vi "Auto_Routine_DepositConeBalance.vi"(8 "error in (no error)":errorcluster, 11 "IsBlue?":bool) -> (0 "error out":errorcluster)   [LabVIEW 2023]
doc: "deposits cone, drives backwards, balances. Starts from 3rd node from non pickup edge. Determines is it is blue or red (by IsBlue?) then changes actions accordingly.\n\ninputs: \n--IsBlue?--Boolean--\n--ErrorIn--\noutputs:\n--ErrorOut--"
uses:
  Arm/ArmGamePiecePreset.ctl
  Arm/ArmPositionPreset.ctl
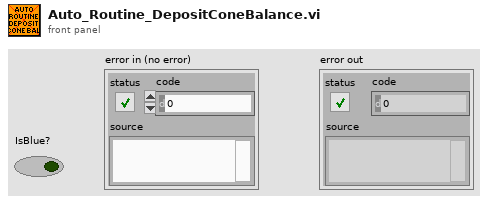
[diagram p1: front panel]
types:
  T1 = typedef "ArmGamePiecePreset.ctl" = enum16{"Cube", "Cone"}
  T2 = typedef "ArmPositionPreset.ctl" = enum16{"Upper", "Lower", "Middle", "Home", "Shelf", "Floor", "HalfFloor", "HalfHome"}
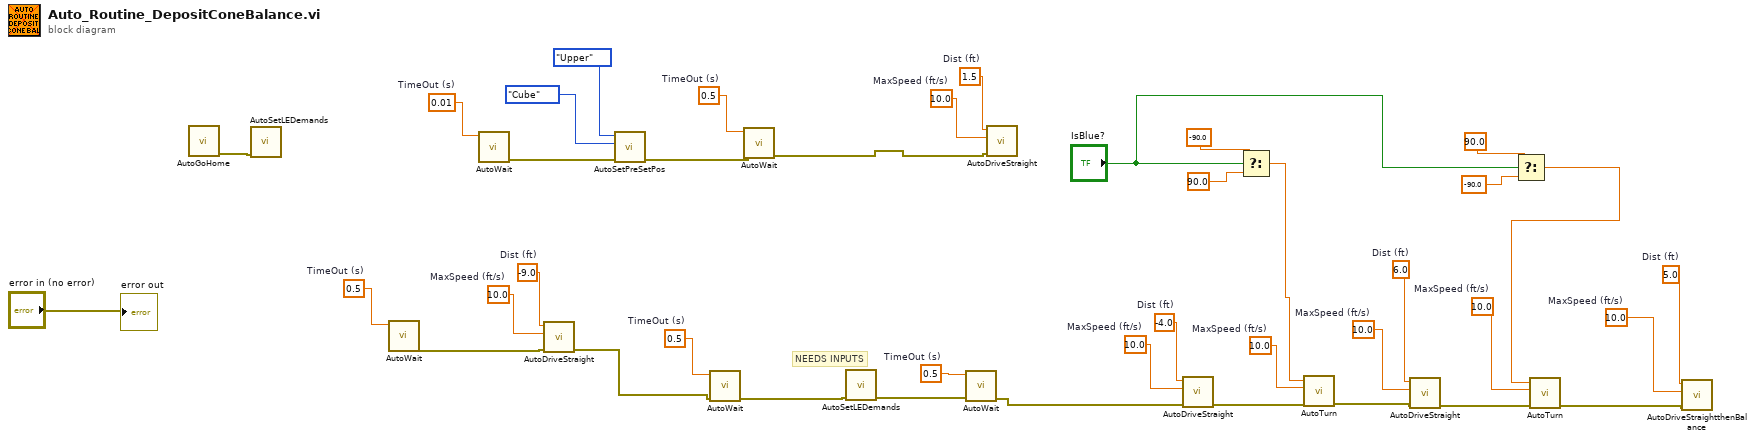
[diagram p0: block diagram]
diagram:
  w14 = 10.0  # MaxSpeed (ft/s)
  w15 = 5.0  # Dist (ft)
  w18 = 10.0  # MaxSpeed (ft/s)
  w19 = 10.0  # MaxSpeed (ft/s)
  w20 = 6.0  # Dist (ft)
  w22 = 10.0  # MaxSpeed (ft/s)
  w24 = -4.0  # Dist (ft)
  w25 = 10.0  # MaxSpeed (ft/s)
  w27 = 0.5  # TimeOut (s)
  w29 = 0.5  # TimeOut (s)
  w31 = -9.0  # Dist (ft)
  w32 = 10.0  # MaxSpeed (ft/s)
  w33 = 0.5  # TimeOut (s)
  w34 = 1.5  # Dist (ft)
  w35 = 10.0  # MaxSpeed (ft/s)
  w37 = 0.5  # TimeOut (s)
  w39 = 0.01  # TimeOut (s)
  # "NEEDS INPUTS"
  n1 = call "AutoGoHome.vi"() -> ("error out"=w1:errorcluster)  [unwired: 11 in]
  n2 = call "AutoSetLEDemands.vi"("error in (no error)"=w1) -> ()  [unwired: 10 in, 1 out]
  n3 = call "AutoWait.vi"("TimeOut (s)"=w33) -> ("error out"=w30:errorcluster)  [unwired: 10 in]
  n4 = call "AutoWait.vi"("TimeOut (s)"=w39) -> ("error out"=w38:errorcluster)  [unwired: 10 in]
  n5 = call "AutoDriveStraight.vi"("error in (no error)"=w30, "MaxSpeed (ft/s)"=w32, "Dist (ft)"=w31) -> ("error out"=w11:errorcluster)  [unwired: 8 in]
  n6 = call "AutoSetPreSetPos.vi"("error in (no error)"=w38, "Game Piece"=ArmGamePiecePreset."Cube", "Position"=ArmPositionPreset."Upper") -> ("error out"=w36:errorcluster)  [unwired: 8 in]
  n7 = call "AutoWait.vi"("error in (no error)"=w11, "TimeOut (s)"=w29) -> ("error out"=w28:errorcluster)  [unwired: 9 in]
  n8 = call "AutoWait.vi"("error in (no error)"=w36, "TimeOut (s)"=w37) -> ("error out"=w10:errorcluster)  [unwired: 9 in]
  n9 = call "AutoSetLEDemands.vi"("error in (no error)"=w28) -> ("error out"=w26:errorcluster)  [unwired: 10 in]
  n10 = call "AutoWait.vi"("error in (no error)"=w26, "TimeOut (s)"=w27) -> ("error out"=w9:errorcluster)  [unwired: 9 in]
  n11 = call "AutoDriveStraight.vi"("error in (no error)"=w10, "MaxSpeed (ft/s)"=w35, "Dist (ft)"=w34) -> ()  [unwired: 8 in, 1 out]
  n12 = call "AutoDriveStraight.vi"("error in (no error)"=w9, "MaxSpeed (ft/s)"=w25, "Dist (ft)"=w24) -> ("error out"=w23:errorcluster)  [unwired: 8 in]
  n13 = Select(t=-90.0, s="IsBlue?", f=90.0) -> (s? t:f=w3:dbl)
  n14 = call "AutoTurn.vi"("error in (no error)"=w23, "MaxSpeed (ft/s)"=w22, "degrees"=w3) -> ("error out"=w21:errorcluster)  [unwired: 8 in]
  n15 = call "AutoDriveStraight.vi"("error in (no error)"=w21, "MaxSpeed (ft/s)"=w19, "Dist (ft)"=w20) -> ("error out"=w17:errorcluster)  [unwired: 8 in]
  n16 = Select(t=90.0, s="IsBlue?", f=-90.0) -> (s? t:f=w4:dbl)
  n17 = call "AutoTurn.vi"("error in (no error)"=w17, "MaxSpeed (ft/s)"=w18, "degrees"=w4) -> ("error out"=w16:errorcluster)  [unwired: 8 in]
  n18 = call "AutoDriveStraightthenBalance.vi"("error in (no error)"=w16, "MaxSpeed (ft/s)"=w14, "Dist (ft)"=w15) -> ()  [unwired: 8 in, 1 out]
  "error out" <- "error in (no error)"
